vi "AMC Local Process.vi"() -> ()   [LabVIEW 2009]
doc: "This example demonstrates how to use the AMC library to implement communication between loops in a single VI."
uses:
  vi.lib/NI/AMC/AMC.lvlib
panel:
  out "Process":bool
  out "Status":string
  in  "Process":bool
  in  "Exit":bool
  in  "State Variables":cluster{"CurrentFile":path}
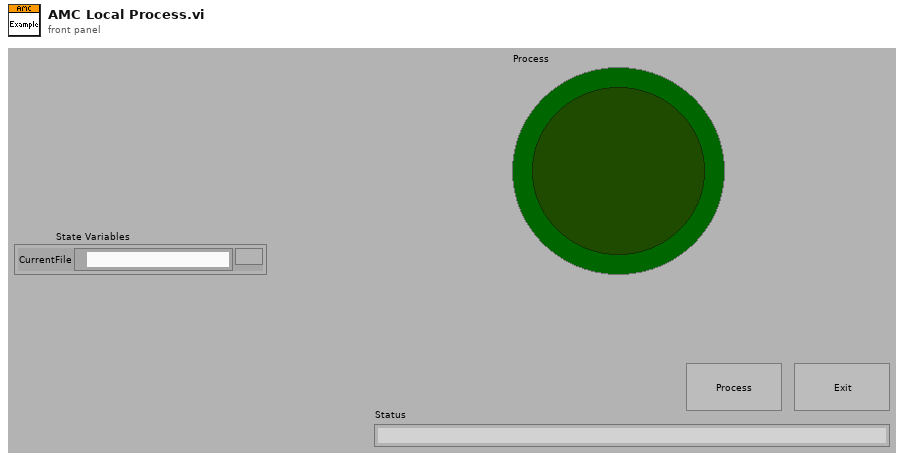
[diagram p1: front panel]
types:
  T1 = typedef "AMC.lvlib/Message Queue.ctl" = refnum<queue>
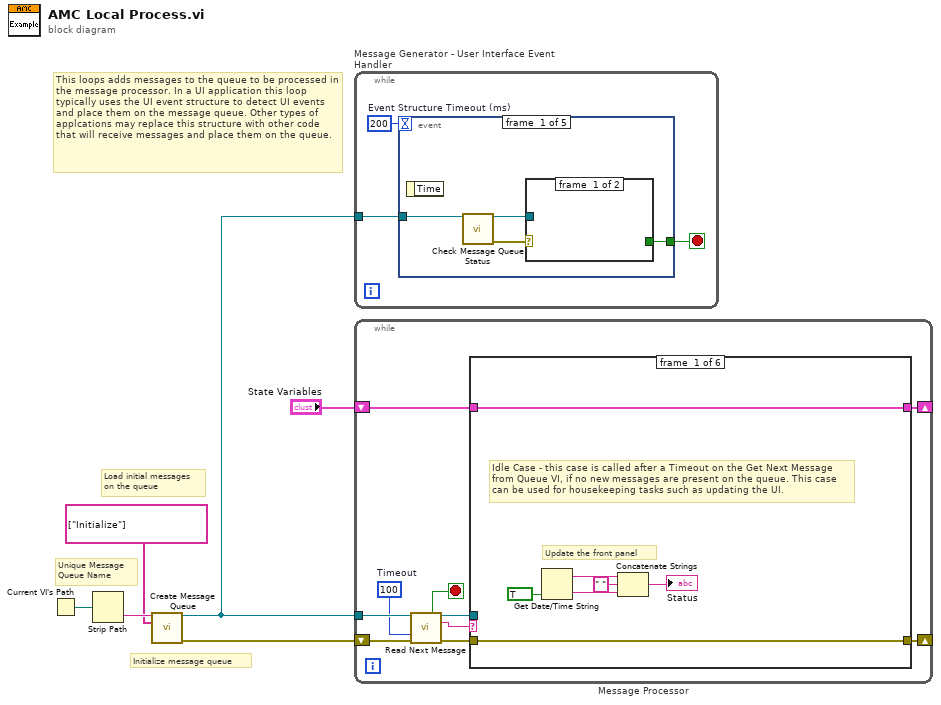
[diagram p0: block diagram]
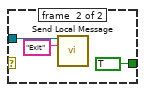
[diagram p2: hidden frame]
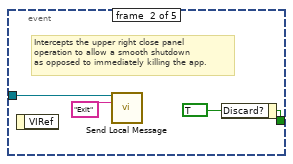
[diagram p3: hidden frame]
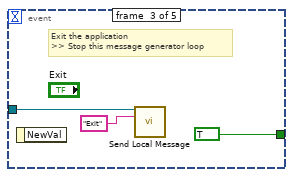
[diagram p4: hidden frame]
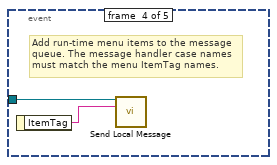
[diagram p5: hidden frame]
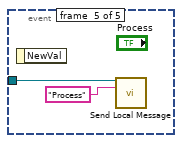
[diagram p6: hidden frame]
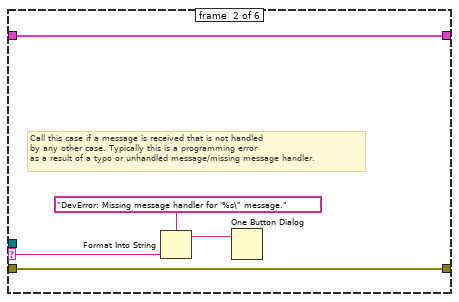
[diagram p7: hidden frame]
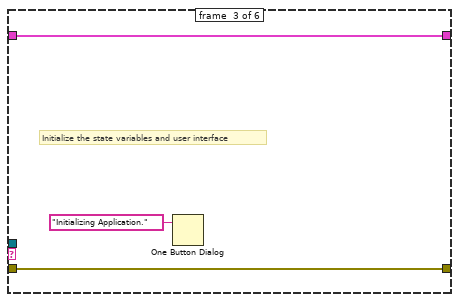
[diagram p8: hidden frame]
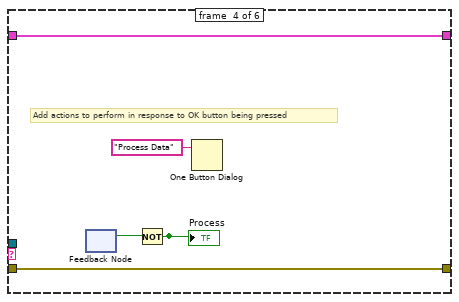
[diagram p9: hidden frame]
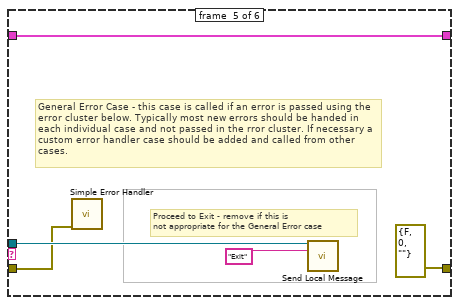
[diagram p10: hidden frame]
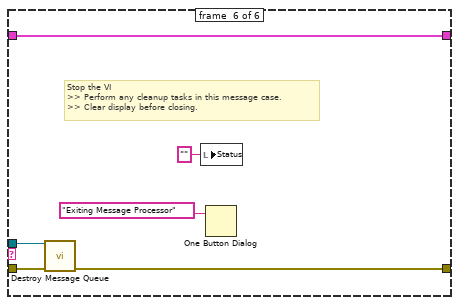
[diagram p11: hidden frame]
diagram:
  # "This loops adds messages to the queue to be processed in the message processor. In a UI application this loop typically uses the UI event structure to detect UI events and place them on the message queue. Other types of applcations may replace this structure with other code that will receive messages and place them on the queue."
  # "Initialize message queue"
  # "Unique Message\nQueue Name"
  # "Load initial messages\non the queue"
  n1 = Current VI's Path() -> (path=w5:path)
  n2 = Strip Path(path=w5) -> (name=w6:string)  [unwired: 1 out]
  n3 = call "Create Message Queue.vi"("message queue name"=w6, "initial message names"=string[] ["Initialize"]) -> ("message queue out"=w4:T1, "error out"=w2:errorcluster)  [unwired: 12 in]
  n4 = while "Message Generator - User Interface Event Handler" {
    tunnel: w4 -> [w7]
    stop <- w8 stop-if-true
    w9 = 200  # Event Structure Timeout (ms)
    n5 = event shown="[2] \"Exit\": Value Change" {
      selector: _ -> [_ _ _ _ _]
      dyn-events: _ -> [_ _ _ _ _]
      timeout: w9 -> [_ _ _ _ _]
      tunnel: [w10 w19 TRUE ("Discard?") _ _] -> w8
      tunnel: w7 -> [w13 w17 w21 w23 w26]
      event #0 {
        n6 = event-data() -> ()  [unwired: 2 out]
        n7 = call "Check Message Queue Status.vi"("message queue in"=w13) -> ("message queue out"=w11:T1, "error out"=w12:errorcluster)  [unwired: 10 in, 3 out]
        n8 = case shown="Error" w12 {
          tunnel: w11 -> [_ w16]
          tunnel: [_ TRUE] -> w10
          frame #0 {
          }
          frame #1 {
            n9 = call "Send Local Message.vi"("message queue in"=w16, "message name"="Exit" ("Message Name")) -> ()  [unwired: 11 in, 3 out]
          }
        }
      }
      event #1 {
        w19 = TRUE ("Discard?")
        # "Intercepts the upper right close panel\noperation to allow a smooth shutdown\nas opposed to immediately killing the app."
        n10 = event-data() -> ()  [unwired: 2 out]
        n11 = call "Send Local Message.vi"("message queue in"=w17, "message name"="Exit") -> ()  [unwired: 11 in, 3 out]
        n12 = event-data("Discard?"=w19) -> ()  [unwired: 1 in, 1 out]
      }
      event #2 {
        # "Exit the application\n>> Stop this message generator loop"
        n13 = event-data() -> ()  [unwired: 2 out]
        n14 = call "Send Local Message.vi"("message queue in"=w21, "message name"="Exit") -> ()  [unwired: 11 in, 3 out]
      }
      event #3 {
        # "Add run-time menu items to the message\nqueue. The message handler case names must match the menu ItemTag names."
        n15 = event-data() -> ("ItemTag"=w24:string)  [unwired: 1 out]
        n16 = call "Send Local Message.vi"("message queue in"=w23, "message name"=w24) -> ()  [unwired: 11 in, 3 out]
      }
      event #4 {
        n17 = event-data() -> ()  [unwired: 2 out]
        n18 = call "Send Local Message.vi"("message queue in"=w26, "message name"="Process") -> ()  [unwired: 11 in, 3 out]
      }
    }
  }
  n19 = while "Message Processor" {
    shift-left: w2 -> [w31]
    shift-right: [w32] -> _
    tunnel: w4 -> [w30]
    shift-left: "State Variables" -> [w36]
    shift-right: [w35] -> _
    stop <- w29 stop-if-true
    w27 = 100  # Timeout
    n20 = call "Read Next Message.vi"("message queue in"=w30, "timeout (1 ms)"=w27, "error in"=w31) -> ("exit process?"=w29:bool, "message queue out"=w34:T1, "message name"=w28:string, "error out"=w33:errorcluster)  [unwired: 5 in, 4 out]
    n21 = case shown="\"Error\"" w28 {
      selector: w28 -> [_ w46 _ _ _ _]
      tunnel: [w43 w48 w51 w55 w61 w66] -> w35
      tunnel: w36 -> [w43 w48 w51 w55 w61 w66]
      tunnel: w34 -> [_ _ _ _ w59 w63]
      tunnel: w33 -> [w42 w47 w50 w56 w58 w67]
      tunnel: [w42 w47 w50 w56 errorcluster {"status"=FALSE, "code"=0, "source"=""} ("error out") w65] -> w32
      frame #0 {
        # "Update the front panel"
        # "Idle Case - this case is called after a Timeout on the Get Next Message from Queue VI, if no new messages are present on the queue. This case can be used for housekeeping tasks such as updating the UI."
        n22 = Get Date/Time String(want seconds? (F)=TRUE) -> (date string=w41:string, time string=w40:string)  [unwired: 2 out]
        n23 = Concatenate Strings(w41, " " ("string"), w40) -> (→"Status":string)
      }
      frame #1 {
        # "Call this case if a message is received that is not handled \nby any other case. Typically this is a programming error\nas a result of a typo or unhandled message/missing message handler."
        n24 = Format Into String(format string="DevError: Missing message handler for '%s\" message." ("message"), w46) -> (resulting string=w44:string)  [unwired: 2 in, 1 out]
        n25 = One Button Dialog(message=w44) -> ()  [unwired: 2 out]
      }
      frame #2 {
        # "Initialize the state variables and user interface"
        n26 = One Button Dialog(message="Initializing Application.") -> ()  [unwired: 2 out]
      }
      frame #3 {
        # "Add actions to perform in response to OK button being pressed"
        n27 = feedback #1() -> (w53:bool)  [unwired: 1 out]
        n28 = Not(x=w53) -> (.not. x?=w52:bool)
        "Process" <- w52
        n29 = One Button Dialog(message="Process Data") -> ()  [unwired: 2 out]
      }
      frame #4 {
        # "Proceed to Exit - remove if this is\nnot appropriate for the General Error case"
        # "General Error Case - this case is called if an error is passed using the error cluster below. Typically most new errors should be handed in each individual case and not passed in the rror cluster. If necessary a custom error handler case should be added and called from other cases."
        n30 = call <vilib>:"Simple Error Handler.vi"("error in (no error)"=w58) -> ()  [unwired: 1 in, 8 out]
        n31 = call "Send Local Message.vi"("message queue in"=w59, "message name"="Exit") -> ()  [unwired: 11 in, 3 out]
      }
      frame #5 {
        # "Stop the VI\n>> Perform any cleanup tasks in this message case.\n>> Clear display before closing."
        n32 = call "Destroy Message Queue.vi"("message queue in"=w63, "error in"=w67) -> ("error out"=w65:errorcluster)  [unwired: 11 in, 2 out]
        n33 = local write "Status"("" ("Status")) -> ()
        n34 = One Button Dialog(message="Exiting Message Processor" ("button name (\"OK\")")) -> ()  [unwired: 2 out]
      }
    }
  }
